vi "Stopwatch.vi"(3 "stop":bool, 11 "OK Button":bool) -> (1 "Elapsed time (seconds)":dbl, 8 "Started":bool, 9 "start time":timestamp)   [LabVIEW 2020]
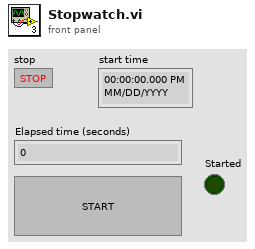
[diagram p1: front panel]
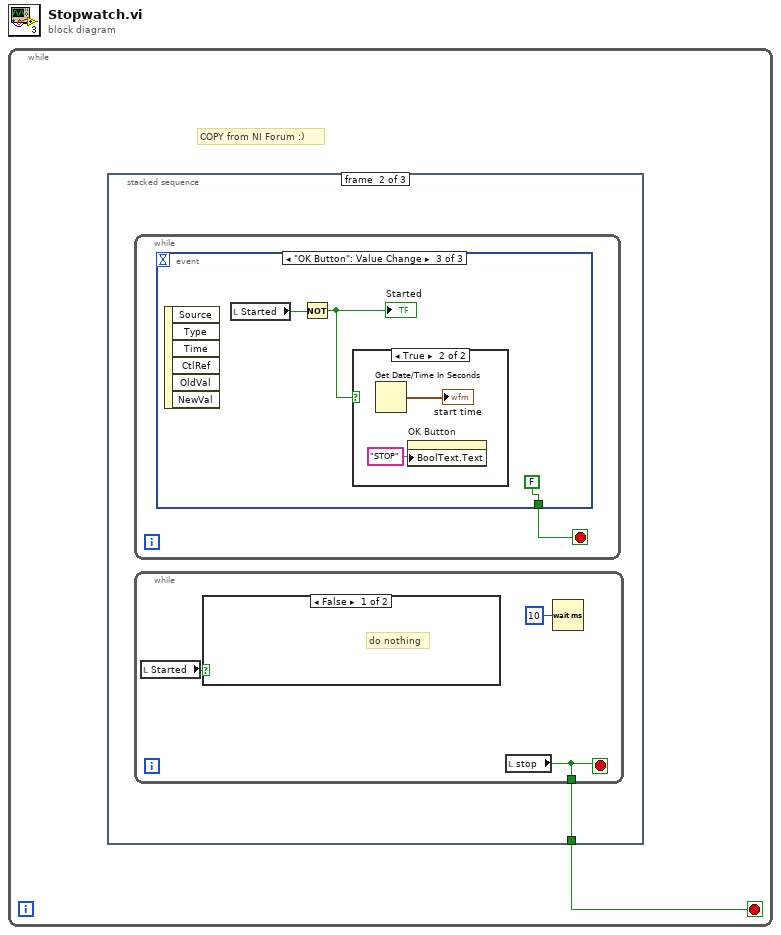
[diagram p0: block diagram]
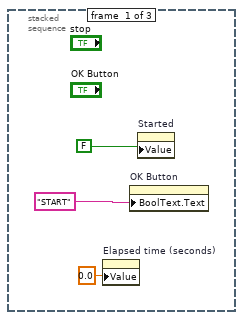
[diagram p2: hidden frame]
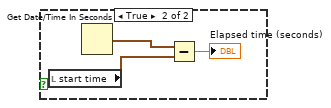
[diagram p3: hidden frame]
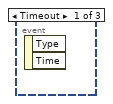
[diagram p4: hidden frame]
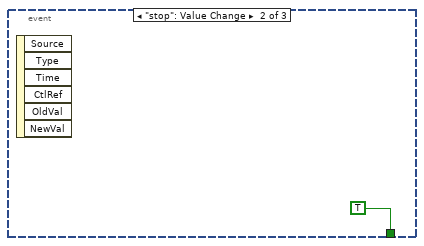
[diagram p5: hidden frame]
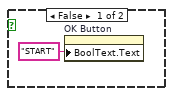
[diagram p6: hidden frame]
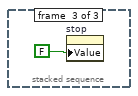
[diagram p7: hidden frame]
diagram:
  n1 = while {
    stop <- w1 stop-if-true
    # "COPY from NI Forum :)"
    n2 = stacked-sequence {
      tunnel: [_ w5 _] -> w1
      frame #0 {
        n3 = property on="Elapsed time (seconds)" class="DigNum (strict)"("Value"=0.0 ("Elapsed time (seconds)")) -> ()  [unwired: 2 in, 2 out]
        n4 = property on="OK Button" class="Bool"("BoolText.Text"="START" ("Caption.Text")) -> ()  [unwired: 2 in, 2 out]
        n5 = property on="Started" class="Bool (strict)"("Value"=FALSE ("Started")) -> ()  [unwired: 2 in, 2 out]
      }
      frame #1 {
        n6 = while {
          stop <- w12 stop-if-true
          n7 = event shown="[2] \"OK Button\": Value Change" {
            selector: _ -> [_ _ _]
            dyn-events: _ -> [_ _ _]
            timeout: _ -> [_ _ _]
            tunnel: [_ TRUE FALSE] -> w12
            event Timeout {
              n8 = event-data() -> ()  [unwired: 1 in, 2 out]
            }
            event "stop": Value Change {
              n9 = event-data() -> ()  [unwired: 1 in, 6 out]
            }
            event "OK Button": Value Change {
              n10 = event-data() -> ()  [unwired: 1 in, 6 out]
              n11 = local read "Started"() -> (w16:bool)
              n12 = Not(x=w16) -> (.not. x?=w14:bool)
              "Started" <- w14
              n13 = case shown="True" w14 {
                frame False {
                  n14 = property on="OK Button" class="Bool"("BoolText.Text"="START" ("Caption.Text")) -> ()  [unwired: 2 in, 2 out]
                }
                frame True {
                  n15 = Get Date/Time In Seconds() -> (seconds since 1Jan1904=→"start time":timestamp)
                  n16 = property on="OK Button" class="Bool"("BoolText.Text"="STOP" ("Caption.Text")) -> ()  [unwired: 2 in, 2 out]
                }
              }
            }
          }
        }
        n17 = while {
          tunnel: [w6] -> w5
          stop <- w6 stop-if-true
          n18 = local read "Started"() -> (w7:bool)
          n19 = case shown="False" w7 {
            frame False {
              # "do nothing"
            }
            frame True {
              n20 = local read "start time"() -> (w11:timestamp)
              n21 = Get Date/Time In Seconds() -> (seconds since 1Jan1904=w10:timestamp)
              n22 = Subtract(x=w10, y=w11) -> (x-y=→"Elapsed time (seconds)":dbl)
            }
          }
          n23 = local read "stop"() -> (w6:bool)
          n24 = Wait (ms)(milliseconds to wait=u32 10) -> ()  [unwired: 1 out]
        }
      }
      frame #2 {
        n25 = property on="stop" class="Bool (strict)"("Value"=FALSE ("stop")) -> ()  [unwired: 2 in, 2 out]
      }
    }
  }
